vi "ziExample-OutPWA_Signalt.vi"() -> ()   [LabVIEW 2009]
doc: "Control a Zurich instrument device via the LabOne Labview API. \nRequirements: Zurich Instruments UHFLI \nThis example retrives Periodic Waveform Analyzer (PWA) data from an UHFLI instrument.\n\n© Zurich Instruments AG, www.zhinst.com\\"
uses:
  <instrlib>/Zurich Instruments LabOne/Public/Data/ziTypePWAWave.ctl
  <instrlib>/Zurich Instruments LabOne/Public/Configure/ziGetValueString.vi
  <instrlib>/Zurich Instruments LabOne/Public/Configure/ziSetValueDoubleArray.vi
  <vilib>/Analysis/2dsp.llb/Real FFT.vi
  <instrlib>/Zurich Instruments LabOne/Public/Data/ziGetEventPWAWave.vi
  <instrlib>/Zurich Instruments LabOne/Zurich Instruments LabOne.lvlib
  <vilib>/Analysis/NI_AALPro.lvlib
  <vilib>/Analysis/NI_AALBase.lvlib
panel:
  out "Error Out":errorcluster
  out "Selected Device":string
  in  "Address":string="DEV"
  in  "Bins":i32=512
  in  "stop":bool
  out "PWAWave":T1={"Timestamp (ticks)"=2149, "SampleCount"=0, "InputSelect"=0, "OscSelect"=0, "Harmonic"=0, "BinCount"=0, "Frequency (Hz)"=0.0, "PWAType"=0, "Mode"=0, "Overflow"=0, "Commensurable"=0, "BinPhase"=[], "X"=[], "Y"=[], "countBin"=[]} {"Frequency (Hz)" format="%#_6p"}
  out "FFT / Harmonics":dbl[](graph)
  out "Waveform":cluster{dbl[], dbl[]}(graph)
  out "Counts per Bin":cluster{dbl[], u32[]}(graph)
  # "ziExample-PWA.vi\nRequirements: UHFLI + BOX +MF\nsee block diagram for VI description"
  # "Tested Devices:\n- UHFLI"
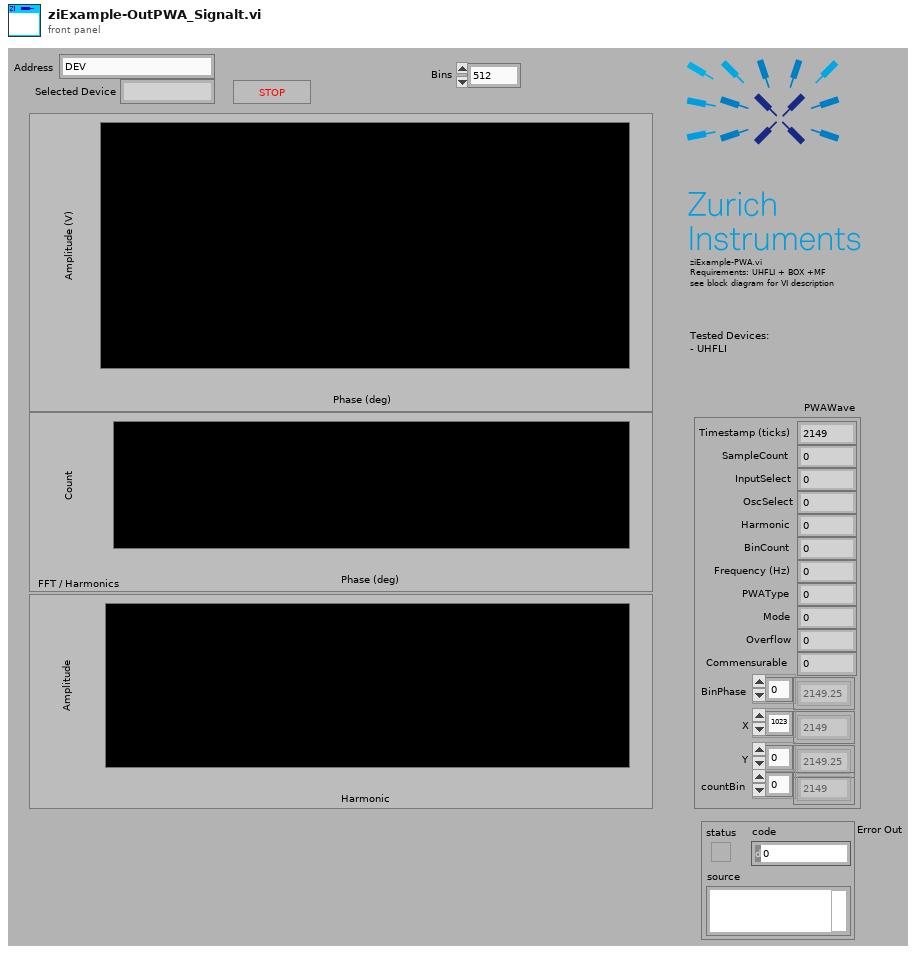
[diagram p1: front panel]
types:
  T1 = typedef "Zurich Instruments LabOne.lvlib/ziTypePWAWave.ctl" = cluster{"Timestamp (ticks)":u64, "SampleCount":u64, "InputSelect":i32, "OscSelect":i32, "Harmonic":i32, "BinCount":i32, "Frequency (Hz)":dbl, "PWAType":u8, "Mode":u8, "Overflow":u8, "Commensurable":u8, "BinPhase":dbl[], "X":dbl[], "Y":dbl[], "countBin":u32[]}
  T2 = typedef "Zurich Instruments LabOne.lvlib/ziTypeHandle.ctl" = cluster{"handleValid":bool, "Conn":u64, "Path Prefix":string, "Handle":u64, "Connected":bool, "Clockbase(s)":dbl}
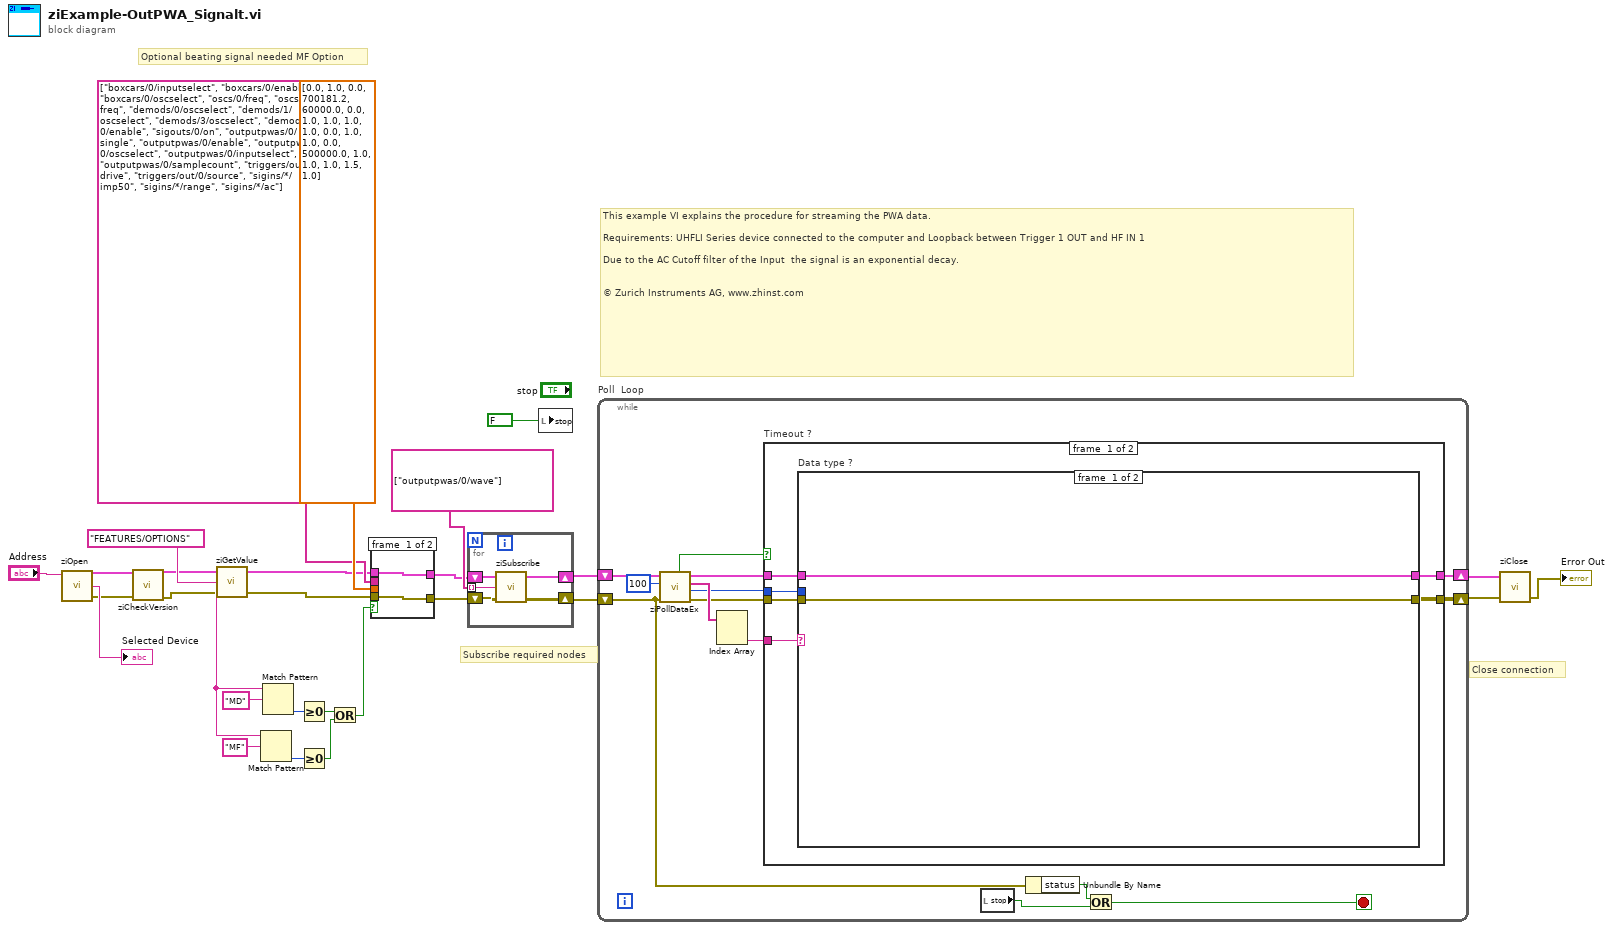
[diagram p0: block diagram]
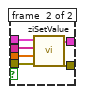
[diagram p2: hidden frame]
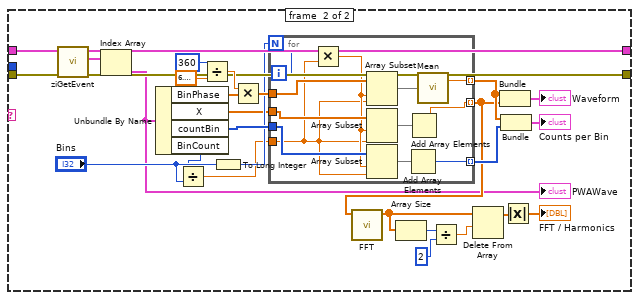
[diagram p3: hidden frame]
diagram:
  # "Optional beating signal needed MF Option"
  # "Close connection"
  # "Subscribe required nodes"
  # "This example VI explains the procedure for streaming the PWA data.\n\nRequirements: UHFLI Series device connected to the computer and Loopback between Trigger 1 OUT and HF IN 1\n\nDue to the AC Cutoff filter of the Input  the signal is an exponential decay.\n\n\n© Zurich Instruments AG, www.zhinst.com"
  n1 = call <instrlib>:"ziOpen.vi"("Address"="Address") -> ("Error Out"=w4:errorcluster, "Selected Device"=→"Selected Device":string, "HandleOut"=w1:T2)  [unwired: 1 in, 2 out]
  n2 = call <instrlib>:"ziCheckVersion.vi"("Handle In"=w1, "Error In"=w4) -> ("Handle Out"=w2:T2, "Error Out"=w3:errorcluster)  [unwired: 11 in, 1 out]
  n3 = call-poly <instrlib>:"ziGetValue.vi"("error in"=w3, "Path"="FEATURES/OPTIONS", "Handle In"=w2) -> ("error out"=w7:errorcluster, "Value"=w12:string, "Handle Out"=w6:T2)
  n4 = Match Pattern(string=w12, regular expression="MF") -> (offset past match=w10:i32)  [unwired: 1 in, 3 out]
  n5 = Match Pattern(string=w12, regular expression="MD") -> (offset past match=w13:i32)  [unwired: 1 in, 3 out]
  n6 = Greater Or Equal To 0?(x=w13) -> (x >= 0?=w9:bool)
  n7 = Greater Or Equal To 0?(x=w10) -> (x >= 0?=w8:bool)
  n8 = Or(x=w9, y=w8) -> (x .or. y?=w5:bool)
  n9 = case shown="True" w5 {
    tunnel: [w30 w36] -> w20
    tunnel: [w29 w35] -> w19
    tunnel: dbl[] [0.0, 1.0, 0.0, 700181.2, 60000.0, 0.0, 1.0, 1.0, 1.0, 1.0, 0.0, 1.0, 1.0, 0.0, 500000.0, 1.0, 1.0, 1.0, 1.5, 1.0] ("abs(x)") -> [_ w34]
    tunnel: string[] ["boxcars/0/inputselect", "boxcars/0/enable", "boxcars/0/oscselect", "oscs/0/freq", "oscs/1/freq", "demods/0/oscselect", "demods/1/oscselect", "demods/3/oscselect", "demods/0/enable", "sigouts/0/on", "outputpwas/0/single", "outputpwas/0/enable", "outputpwas/0/oscselect", "outputpwas/0/inputselect", "outputpwas/0/samplecount", "triggers/out/0/drive", "triggers/out/0/source", "sigins/*/imp50", "sigins/*/range", "sigins/*/ac"] -> [_ w33]
    tunnel: w7 -> [w29 w32]
    tunnel: w6 -> [w30 w31]
    frame #0 {
    }
    frame #1 {
      n10 = call-poly <instrlib>:"ziSetValue.vi"("Error In"=w32, "Values"=w34, "Paths"=w33, "Handle In"=w31) -> ("Error Out"=w35:errorcluster, "Handle Out"=w36:T2)  [unwired: 1 in]
    }
  }
  n11 = for {
    shift-right: [w41] -> w24
    shift-left: w20 -> [w39]
    shift-right: [w40] -> w23
    shift-left: w19 -> [w38]
    tunnel: string[] ["outputpwas/0/wave"] -> [w37] mode=indexing
    n12 = call <instrlib>:"ziSubscribe.vi"("error in"=w38, "Path ()"=w37, "Handle In"=w39) -> ("error out"=w40:errorcluster, "Handle Out"=w41:T2)  [unwired: 1 in]
  }
  n13 = local write "stop"(FALSE ("Record")) -> ()
  n14 = while "Poll  Loop" {
    shift-right: [w48] -> w25
    shift-left: w24 -> [w55]
    shift-right: [w46] -> w26
    shift-left: w23 -> [w44]
    stop <- w42 stop-if-true
    n15 = call <instrlib>:"ziPollDataEx.vi"("error in"=w44, "Timeout ms (50)"=100 ("TimeOut ms (50)"), "Handle In"=w55) -> ("error out"=w47:errorcluster, "Timestamp (ticks)"=w50:u64, "PathArray"=w52:string[], "Handle Out"=w49:T2, "Timed Out"=w53:bool)  [unwired: 1 in, 3 out]
    n16 = Index Array(array=w52) -> (element #2=w51:string)  [unwired: 2 in, 1 out]
    n17 = case "Timeout ?" shown="False" w53 {
      tunnel: w51 -> [w61 _]
      tunnel: w50 -> [w60 _]
      tunnel: w49 -> [w59 w105]
      tunnel: [w58 w105] -> w48
      tunnel: w47 -> [w57 w104]
      tunnel: [w56 w104] -> w46
      frame #0 {
        n18 = case "Data type ?" shown="\"OUTPUTPWAS\"" w61 {
          tunnel: w60 -> [_ _]
          tunnel: w59 -> [w63 w91]
          tunnel: [w63 w90] -> w58
          tunnel: w57 -> [w62 w78]
          tunnel: [w62 w77] -> w56
          frame #0 {
          }
          frame #1 {
            n19 = call-poly <instrlib>:"ziGetEvent.vi"("Error In"=w78, "Handle In"=w91) -> ("Error Out"=w77:errorcluster, "PWAWaves Out"=w76:T1[], "Handle Out"=w90:T2)  [unwired: 7 in]
            n20 = Index Array(array=w76) -> (element=w67:T1)  [unwired: 1 in]
            "PWAWave" <- w67
            n21 = Unbundle By Name(w67) -> ("BinPhase"=w65:dbl[], "X"=w66:dbl[], "countBin"=w89:u32[], "BinCount"=w64:i32)
            n22 = Divide(x=w64, y="Bins") -> (x/y=w69:dbl)
            n23 = Divide(x=360, y=6.283185307179586) -> (x/y=w86:dbl)
            n24 = To Long Integer(number="Bins") -> (32bit integer=w71:i32)
            n25 = Multiply(x=w86, y=w65) -> (x*y=w85:dbl[])
            n26 = for {
              N: w71 -> [_]
              tunnel: w89 -> [w101]
              tunnel: w85 -> [w103]
              tunnel: w66 -> [w97]
              tunnel: w69 -> [w95]
              tunnel: [w93] -> w75 mode=indexing
              tunnel: [w98] -> w74 mode=indexing
              tunnel: [w92] -> w68 mode=indexing
              i -> [w102]
              n27 = Multiply(x=w102, y=w95) -> (x*y=w96:dbl)
              n28 = Array Subset(array=w103, index=w96, length=w95) -> (w99:dbl[])
              n29 = Array Subset(array=w97, index=w96, length=w95) -> (w94:dbl[])
              n30 = Array Subset(array=w101, index=w96, length=w95) -> (w100:u32[])
              n31 = Add Array Elements(numeric array=w100) -> (sum=w93:u32)
              n32 = Add Array Elements(numeric array=w94) -> (sum=w92:dbl)
              n33 = call <vilib>:"Mean.vi"("X"=w99) -> ("mean"=w98:dbl)  [unwired: 1 out]
            }
            n34 = call-poly <vilib>:"FFT.vi"("X"=w68) -> ("FFT {X}"=w82:cdb[])  [unwired: 9 in, 1 out]
            n35 = Array Size(array=w82) -> (size(s)=w81:i32)
            n36 = Divide(x=w81, y=2) -> (x/y=w79:dbl)
            n37 = Delete From Array(array=w82, length=w79) -> (array with subset deleted=w83:cdb[])  [unwired: 1 in, 1 out]
            n38 = Bundle(w74, w68) -> (→"Waveform":cluster{dbl[], dbl[]})  [unwired: 1 in]
            n39 = Bundle(w74, w75) -> (→"Counts per Bin":cluster{dbl[], u32[]})  [unwired: 1 in]
            n40 = Absolute Value(x=w83) -> (abs(x)=→"FFT / Harmonics":dbl[])
          }
        }
      }
      frame #1 {
        # "Timeout, no action."
      }
    }
    n41 = local read "stop"() -> (w43:bool)
    n42 = Unbundle By Name(w44) -> ("status"=w45:bool)
    n43 = Or(x=w45, y=w43) -> (x .or. y?=w42:bool)
  }
  n44 = call <instrlib>:"ziClose.vi"("Error In"=w26, "Handle In"=w25) -> ("Error Out"=→"Error Out":errorcluster)  [unwired: 3 out]
